vi "流程写入.vi"(11 "添加的路径":path) -> ()   [LabVIEW 2016, in "斯坦道CODCr.lvlib"]
uses:
  <vilib>/Utility/miscctls.llb/LVPointTypeDef.ctl
panel:
  in  "选项卡控件":enum32{"测试流程", "简易流程"}(tab)
  in  "一键写入":bool
  in  "量程下拉列表":enum16{"低量程", "高量程"}(ring)
  in  "测量模式":T1(ring)
  in  "简易流程":u16(ring)
  in  "一键写入 2":bool=TRUE
  in  "关闭":bool
  out "字符串":string
  in  "写入":bool
  in  "参数下拉列表":u16(ring) items=["总氮"=1, "总磷"=2]
  # "请选择要写入的流程"
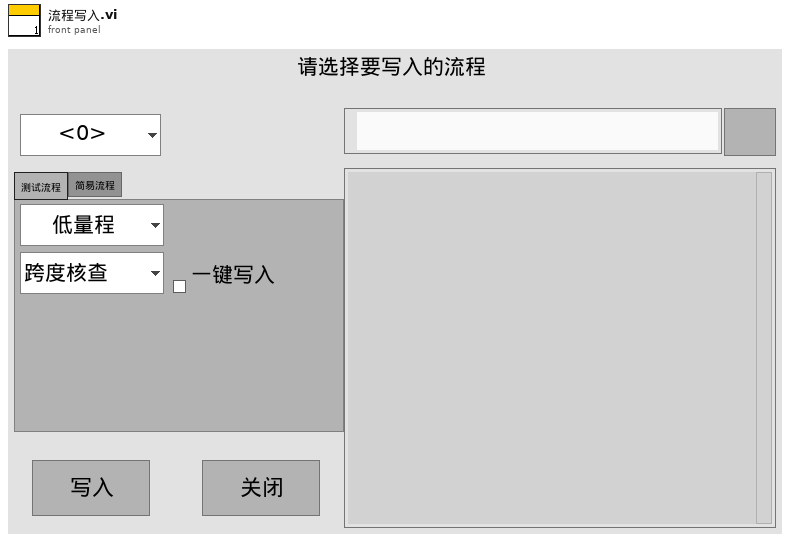
[diagram p1: front panel]
types:
  T1 = enum16{"跨度核查", "水样测量", "零点核查", "标样核查", "加标回收", "快捷测试", "空白校准", "标样校准"}
  T2 = typedef "LVPointTypeDef.ctl" = cluster{"Horizontal":i16, "Vertical":i16}
  T3 = typedef "LVStringsAndValuesArrayTypeDef_U16.ctl" = cluster{"String":string, "Value":u16}[]
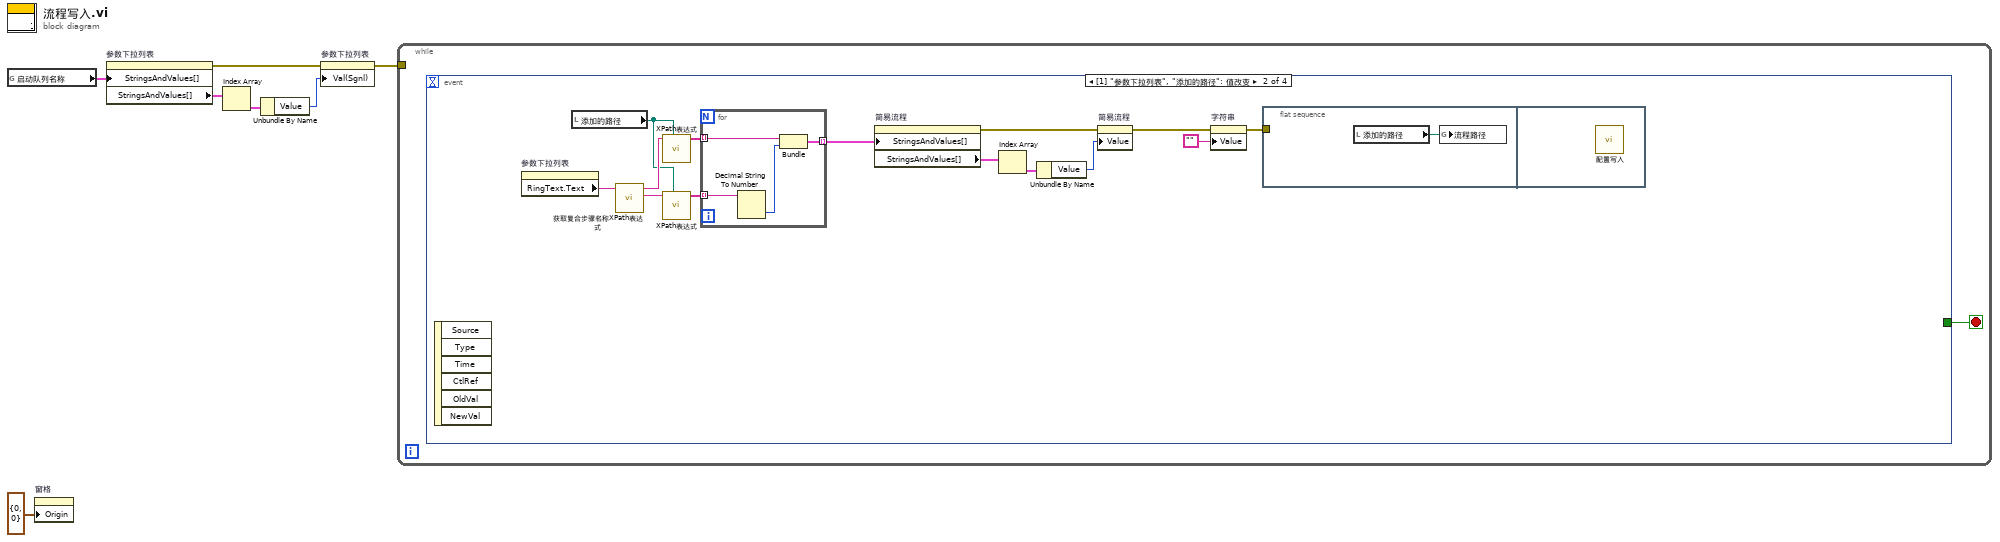
[diagram p0: block diagram]
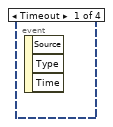
[diagram p2: hidden frame]
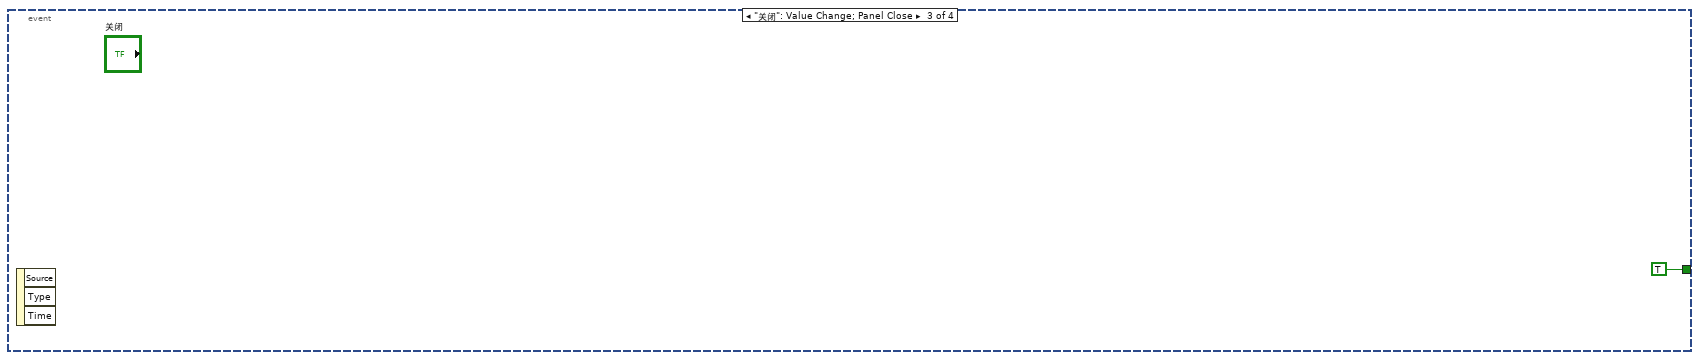
[diagram p3: hidden frame]
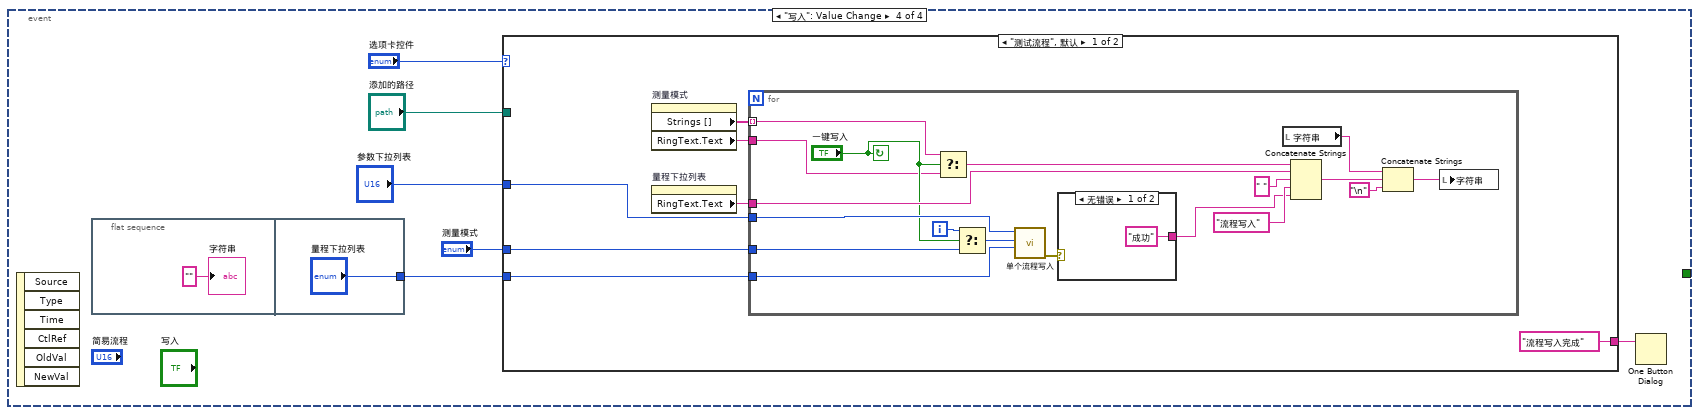
[diagram p4: hidden frame]
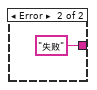
[diagram p5: hidden frame]
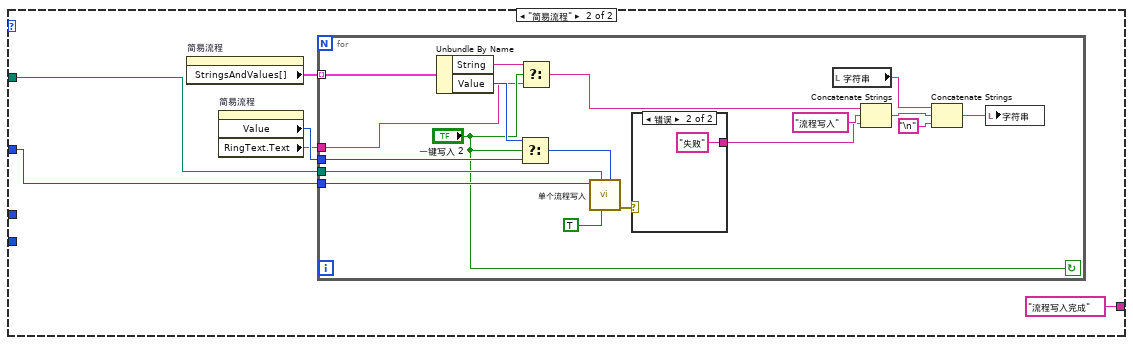
[diagram p6: hidden frame]
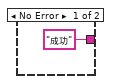
[diagram p7: hidden frame]
diagram:
  n1 = global read "总磷总氮断电保存全局变量.vi" "启动队列名称"() -> (w6:cluster{"String":string, "Value":u16}[])
  n2 = property on="窗格" class="Pane"("Origin"=T2 {"Horizontal"=0, "Vertical"=0} ("原点")) -> ()  [unwired: 2 in, 2 out]
  n3 = property on="参数下拉列表" class="Ring (严格)"("StringsAndValues[]"=w6) -> (error out=w5:errorcluster, "StringsAndValues[]"=w4:T3)  [unwired: 2 in, 1 out]
  n4 = Index Array(array=w4) -> (element=w3:cluster{"String":string, "Value":u16})  [unwired: 1 in]
  n5 = Unbundle By Name(w3) -> ("Value"=w2:u16)
  n6 = property on="参数下拉列表" class="Ring (严格)"(error in=w5, "Val(Sgnl)"=w2) -> (error out=w1:errorcluster)  [unwired: 1 in, 1 out]
  n7 = while {
    tunnel: w1 -> [_]
    stop <- w8 stop-if-true
    n8 = event shown="[1] \"参数下拉列表\", \"添加的路径\": 值改变" {
      selector: _ -> [_ _ _ _]
      dyn-events: _ -> [_ _ _ _]
      timeout: _ -> [_ _ _ _]
      tunnel: [_ _ TRUE _] -> w8
      event Timeout {
        n9 = event-data() -> ()  [unwired: 1 in, 3 out]
      }
      event "参数下拉列表", "添加的路径": Value Change {
        n10 = event-data() -> ()  [unwired: 1 in, 6 out]
        n11 = property on="参数下拉列表" class="Ring (严格)"() -> ("RingText.Text"=w21:string)  [unwired: 2 in, 2 out]
        n12 = local read "添加的路径"() -> (w20:path)
        n13 = call "获取复合步骤名称XPath表达式.vi"("查询参数"=w21) -> ("FlowId"=w19:string, "name"=w22:string)  [unwired: 9 in]
        n14 = call "XPath表达式.vi"("添加的路径"=w20, "XPath expression"=w22) -> ("数组"=w18:string[])  [unwired: 9 in]
        n15 = call "XPath表达式.vi"("添加的路径"=w20, "XPath expression"=w19) -> ("数组"=w17:string[])  [unwired: 9 in]
        n16 = for {
          tunnel: w18 -> [w27] mode=indexing
          tunnel: w17 -> [w26] mode=indexing
          tunnel: [w24] -> w16 mode=indexing
          n17 = Decimal String To Number(string=w26) -> (number=w25:i32)  [unwired: 2 in, 1 out]
          n18 = Bundle("node text"=w27, w25) -> (w24:cluster{"node text":string, i32})  [unwired: 1 in]
        }
        n19 = property on="简易流程" class="Ring (严格)"("StringsAndValues[]"=w16) -> (error out=w15:errorcluster, "StringsAndValues[]"=w14:T3)  [unwired: 2 in, 1 out]
        n20 = Index Array(array=w14) -> (element=w13:cluster{"String":string, "Value":u16})  [unwired: 1 in]
        n21 = Unbundle By Name(w13) -> ("Value"=w12:u16)
        n22 = property on="简易流程" class="Ring (严格)"(error in=w15, "Value"=w12) -> (error out=w11:errorcluster)  [unwired: 1 in, 1 out]
        n23 = property on="字符串" class="Str"(error in=w11, "Value"="") -> (error out=w9:errorcluster)  [unwired: 1 in, 1 out]
        n24 = flat-sequence {
          tunnel: w9 -> [_]
          frame #0 {
            n25 = local read "添加的路径"() -> (w23:path)
            n26 = global write "总磷总氮断电保存全局变量.vi" "流程路径"(w23) -> ()
          }
          frame #1 {
            n27 = call "配置写入.vi"() -> ()  [unwired: 11 in, 1 out]
          }
        }
      }
      event "关闭": Value Change; Panel Close {
        n28 = event-data() -> ()  [unwired: 1 in, 3 out]
      }
      event "写入": Value Change {
        n29 = event-data() -> ()  [unwired: 1 in, 6 out]
        n30 = flat-sequence {
          tunnel: ["量程下拉列表"] -> w33
          frame #0 {
            "字符串" <- ""
          }
          frame #1 {
          }
        }
        n31 = case shown="\"测试流程\", 默认" "选项卡控件" {
          tunnel: "参数下拉列表" -> [w39 w66]
          tunnel: w33 -> [w40 _]
          tunnel: "添加的路径" -> [_ w67]
          tunnel: ["流程写入完成" ("消息") "流程写入完成" ("消息")] -> w30
          tunnel: "测量模式" -> [w37 _]
          frame "测试流程", Default {
            n32 = property on="测量模式" class="Enum (严格)"() -> ("Strings []"=w38:string[], "RingText.Text"=w35:string)  [unwired: 2 in, 2 out]
            n33 = property on="量程下拉列表" class="Enum (严格)"() -> ("RingText.Text"=w36:string)  [unwired: 2 in, 2 out]
            n34 = for {
              tunnel: w40 -> [w52]
              tunnel: w39 -> [w50]
              tunnel: w38 -> [w44] mode=indexing
              tunnel: w37 -> [w49]
              tunnel: w36 -> [w47]
              tunnel: w35 -> [w43]
              i -> [w51]
              stop <- "一键写入" continue-if-true
              n35 = Select(t=w44, s="一键写入", f=w43) -> (s? t:f=w42:string)
              n36 = Select(t=w51, s="一键写入", f=w49) -> (s? t:f=w48:i32)
              n37 = call "单个流程写入.vi"("量程"=w52, "测量模式"=w48, "测量参数"=w50) -> ("error out"=w59:errorcluster)  [unwired: 7 in, 1 out]
              n38 = case shown="无错误" w59 {
                tunnel: ["成功" "失败"] -> w56
                frame No Error {
                }
                frame Error {
                }
              }
              n39 = local read "字符串"() -> (w58:string)
              n40 = Concatenate Strings(w42, w47, " " ("字符串"), "流程写入", w56) -> (w55:string)
              n41 = Concatenate Strings(w58, w55, "\n") -> (w53:string)
              n42 = local write "字符串"(w53) -> ()
            }
          }
          frame "简易流程" {
            n43 = property on="简易流程" class="Ring (严格)"() -> ("StringsAndValues[]"=w65:T3)  [unwired: 2 in, 2 out]
            n44 = property on="简易流程" class="Ring (严格)"() -> ("Value"=w63:u16, "RingText.Text"=w62:string)  [unwired: 2 in, 2 out]
            n45 = for {
              tunnel: w65 -> [w75] mode=indexing
              tunnel: w67 -> [w78]
              tunnel: w66 -> [w77]
              tunnel: w63 -> [w72]
              tunnel: w62 -> [w69]
              stop <- "一键写入 2" continue-if-true
              n46 = Unbundle By Name(w75) -> ("String"=w70:string, "Value"=w74:u16)
              n47 = Select(t=w74, s="一键写入 2", f=w72) -> (s? t:f=w73:u16)
              n48 = Select(t=w70, s="一键写入 2", f=w69) -> (s? t:f=w68:string)
              n49 = call "单个流程写入.vi"("简易流程Id"=w73, "是否是简易流程"=TRUE, "添加的路径"=w78, "测量参数"=w77) -> ("error out"=w85:errorcluster)  [unwired: 6 in, 1 out]
              n50 = case shown="错误" w85 {
                tunnel: ["成功" "失败"] -> w82
                frame No Error {
                }
                frame Error {
                }
              }
              n51 = local read "字符串"() -> (w84:string)
              n52 = Concatenate Strings(w68, "流程写入", w82) -> (w81:string)
              n53 = Concatenate Strings(w84, w81, "\n") -> (w79:string)
              n54 = local write "字符串"(w79) -> ()
            }
          }
        }
        n55 = One Button Dialog(message=w30) -> ()  [unwired: 1 in, 1 out]
      }
    }
  }
